vi "Get all divisors-power set.vi"(8 "error in (no error)":errorcluster, 10 "Sort output divisors? (dflt=FALSE)":bool, 11 "x":i32) -> (0 "error out":errorcluster, 1 "Execution time (ms)-Total":u32, 2 "no. of divisors":i32, 3 "Divisors":i32[](array[numeric]))   [LabVIEW 2021, in "Numeric Utilities.lvlib"]
uses:
  Numeric Utilities.lvlib
  Factors cluster.ctl
  <userlib>/_OpenG.lib/array/array.llb/Index 1D Array Elements (I32)__ogtk.vi
  <userlib>/_OpenG.lib/array/array.llb/Remove Duplicates from 1D Array (I32)__ogtk.vi
  Named Timers/Named Timers.lvlib
panel:
  out "Execution time (ms)-power set":u32
  out "no. of spread out factors":i32
  out "no. of subsets":i32
  out "Factors":T1[](array[typedef])
  out "prime factors (spread out)":i32[](array[numeric])
  # "Development\ncontrols/indicators useful for development and testing, but which are not outputs of the VI"
  # "Input\nInputs to the VI"
  # "Output\nOutputs of the VI"
  # "Description\n\nBlank VI with error handling case. \n\nSummarize the use of this VI in this space."
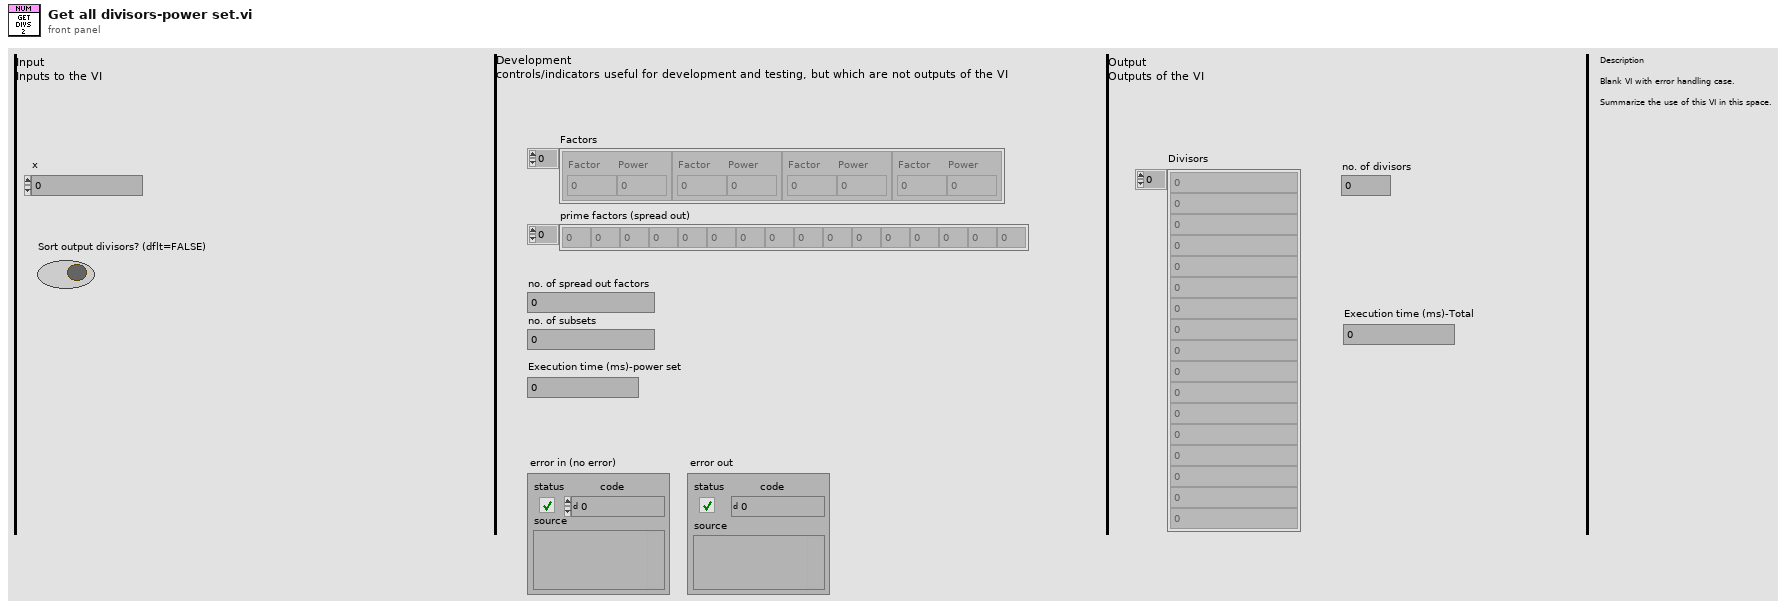
[diagram p1: front panel]
types:
  T1 = typedef "Numeric Utilities.lvlib/Factors cluster.ctl" = cluster{"Factor":i32, "Power":i32}
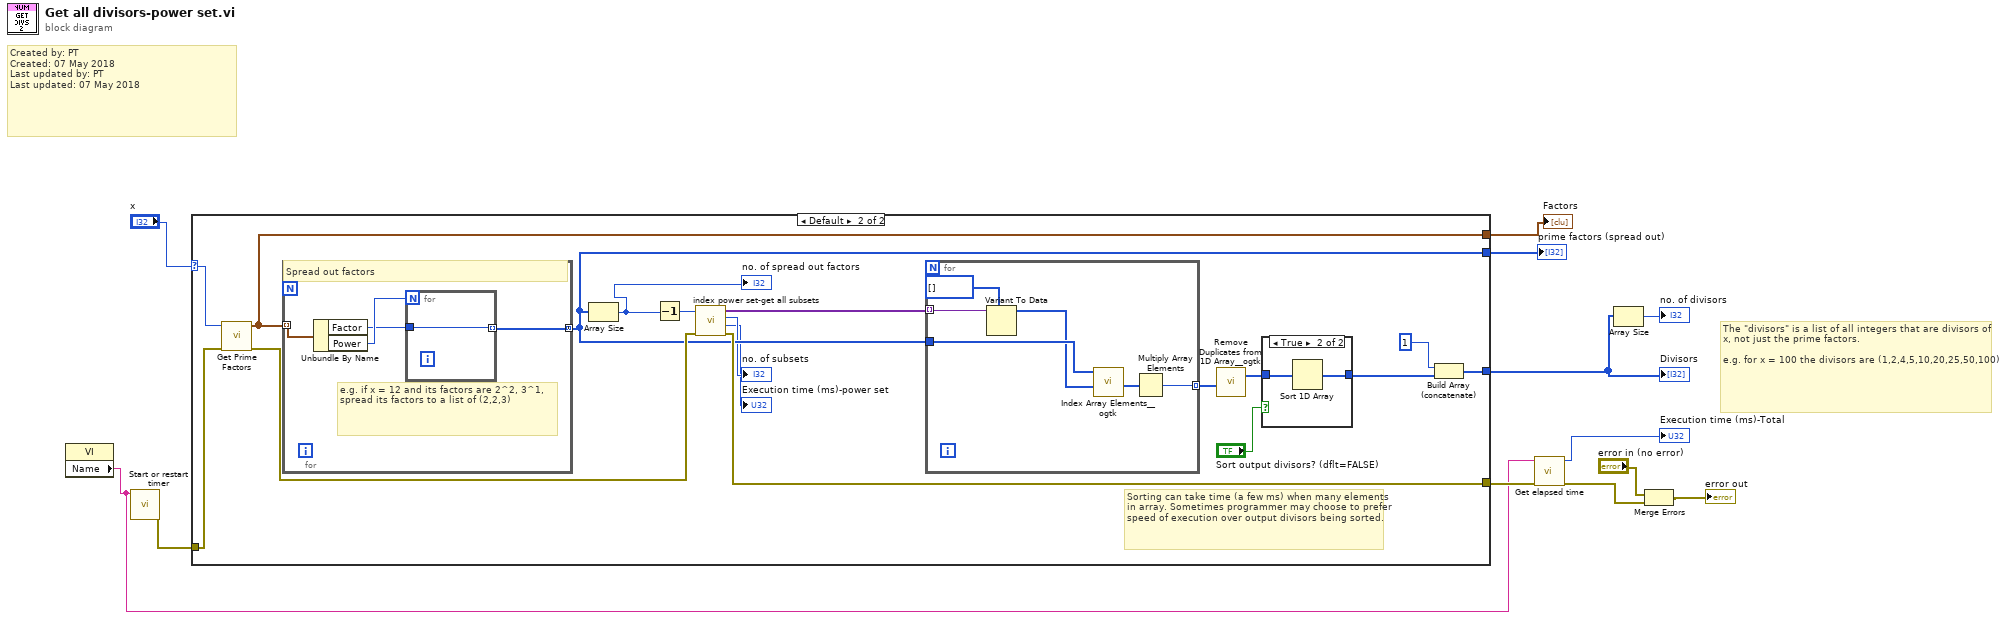
[diagram p0: block diagram]
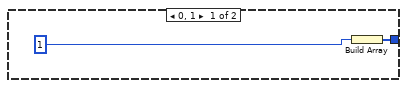
[diagram p2: hidden frame]
diagram:
  # "The \"divisors\" is a list of all integers that are divisors of x, not just the prime factors.\n\ne.g. for x = 100 the divisors are (1,2,4,5,10,20,25,50,100)"
  # "Created by: PT\nCreated: 07 May 2018\nLast updated by: PT\nLast updated: 07 May 2018"
  n1 = property class="VI"() -> ("Name"=w3:string)  [unwired: 2 in, 2 out]
  n2 = call "Start or restart timer.vi"("Timer name"=w3) -> ("error out"=w5:errorcluster)  [unwired: 10 in]
  n3 = case shown="Default" "x" {
    selector: "x" -> [_ w24]
    tunnel: [w13 w26] -> w11
    tunnel: [_ w19] -> w9
    tunnel: [_ w22] -> w6
    tunnel: w5 -> [_ w21]
    tunnel: [_ w20] -> w1
    frame 0, 1 {
      n4 = Build Array(1) -> (w13:i32[])
    }
    frame Default {
      # "Sorting can take time (a few ms) when many elements in array. Sometimes programmer may choose to prefer speed of execution over output divisors being sorted."
      n5 = call "Get Prime Factors.vi"("error in (no error)"=w21, "x"=w24) -> ("error out"=w23:errorcluster, "Factors out"=w20:T1[])  [unwired: 4 in, 4 out]
      n6 = for {
        tunnel: w20 -> [w44] mode=indexing
        tunnel: [w41] -> w19 mode=concatenating
        # "e.g. if x = 12 and its factors are 2^2, 3^1, spread its factors to a list of (2,2,3)"
        # "Spread out factors"
        n7 = Unbundle By Name(w44) -> ("Factor"=w42:i32, "Power"=w43:i32)
        n8 = for {
          N: w43 -> [_]
          tunnel: w42 -> [w45]
          tunnel: [w45] -> w41 mode=indexing
        }
      }
      n9 = Array Size(array=w19) -> (size(s)=w17:i32)
      "no. of spread out factors" <- w17
      n10 = Decrement(x=w17) -> (x-1=w31:i32)
      n11 = call "index power set-get all subsets.vi"("error in (no error)"=w23, "End index"=w31) -> ("error out"=w22:errorcluster, "Execution time (ms)"=→"Execution time (ms)-power set":u32, "no. of subsets"=→"no. of subsets":i32, "Subsets of indexes"=w30:variant[])  [unwired: 6 in]
      n12 = for {
        tunnel: w30 -> [w40] mode=indexing
        tunnel: w19 -> [w38]
        tunnel: [w35] -> w29 mode=indexing
        n13 = Variant To Data(type=i32[] [], Variant=w40) -> (data=w37:i32[])  [unwired: 1 in, 1 out]
        n14 = call-poly <userlib>:"Index Array Elements__ogtk.vi"("indices"=w37, "array"=w38) -> ("elements"=w36:i32[])  [unwired: 9 in]
        n15 = Multiply Array Elements(1:w36) -> (0:w35:i32)
      }
      n16 = call-poly <userlib>:"Remove Duplicates from 1D Array__ogtk.vi"("Input Array"=w29) -> ("Output Array"=w28:i32[])  [unwired: 1 out]
      n17 = case shown="True" "Sort output divisors? (dflt=FALSE)" {
        tunnel: w28 -> [w32 w34]
        tunnel: [w32 w33] -> w27
        frame False {
        }
        frame True {
          n18 = Sort 1D Array(array=w34) -> (sorted array=w33:i32[])
        }
      }
      n19 = Build Array (concatenate)(1, w27) -> (w26:i32[])
    }
  }
  "Divisors" <- w11
  "prime factors (spread out)" <- w9
  "Factors" <- w1
  n20 = call "Get elapsed time.vi"("error in (no error)"=w6, "Timer name"=w3) -> ("error out"=w4:errorcluster, "Elapsed time (ms)"=→"Execution time (ms)-Total":u32)  [unwired: 6 in, 2 out]
  n21 = Array Size(array=w11) -> (size(s)=→"no. of divisors":i32)
  n22 = Merge Errors("error in (no error)", w4) -> (→"error out":errorcluster)
